vi "Joystick breakout clean.vi"(0 "Joystick":T3) -> (4 "Axis":T2, 6 "Buttons":T1)   [LabVIEW 2014]
uses:
  <vilib>/Rock Robotics/WPI/Joystick/WPI_JoystickDevRef.ctl
  <vilib>/Rock Robotics/WPI/Joystick/WPI_JoystickDeviceEnum.ctl
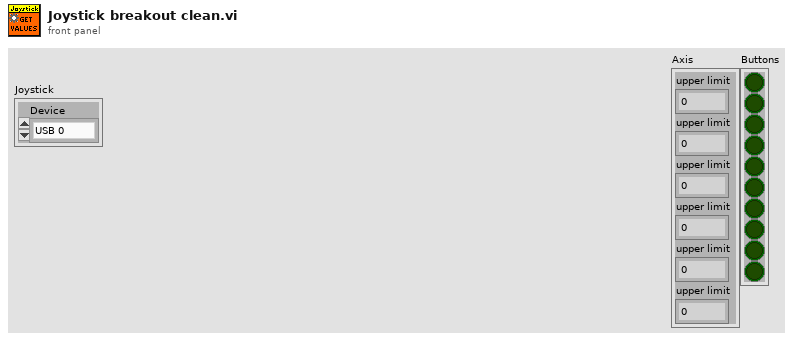
[diagram p1: front panel]
types:
  T1 = cluster{bool, bool, bool, bool, bool, bool, bool, bool, bool, bool}
  T2 = cluster{"upper limit":dbl, "upper limit":dbl, "upper limit":dbl, "upper limit":dbl, "upper limit":dbl, "upper limit":dbl}
  T3 = typedef "WPI_JoystickDevRef.ctl" = cluster{"Device":T4}
  T4 = typedef "WPI_JoystickDeviceEnum.ctl" = enum16{"USB 0", "USB 1", "USB 2", "USB 3", "USB 4", "USB 5"}
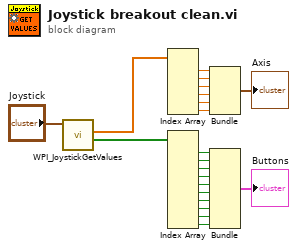
[diagram p0: block diagram]
diagram:
  n1 = call <vilib>:"WPI_JoystickGetValues.vi"("JoystickDevRef"="Joystick") -> ("Buttons"=w19:bool[], "Axes"=w20:dbl[])  [unwired: 6 in, 3 out]
  n2 = Index Array(array=w20) -> (element #1=w13:dbl, element #2=w14:dbl, element #3=w15:dbl, element #4=w16:dbl, element #5=w17:dbl, element #6=w18:dbl)  [unwired: 6 in]
  n3 = Index Array(array=w19) -> (element #1=w11:bool, element #2=w10:bool, element #3=w9:bool, element #4=w8:bool, element #5=w7:bool, element #6=w6:bool, element #7=w5:bool, element #8=w4:bool, element #9=w3:bool, element #10=w2:bool)  [unwired: 10 in]
  n4 = Bundle("upper limit"=w13, "upper limit"=w14, "upper limit"=w15, "upper limit"=w16, "upper limit"=w17, "upper limit"=w18) -> (→"Axis":T2)  [unwired: 1 in]
  n5 = Bundle(w11, w10, w9, w8, w7, w6, w5, w4, w3, w2) -> (→"Buttons":T1)  [unwired: 1 in]
